vi "_Update A Key Value.vi"(4 "error in (no error)":errorcluster, 5 "Value":string="test Key", 6 "Key":string="Key", 7 "node in":refnum<k20>) -> (0 "error out":errorcluster, 3 "node out":refnum<k20>)   [LabVIEW 2012]
uses:
  <vilib>/xml/Close Reference(Node).vi
  <vilib>/xml/NI_XML.lvlib
  <resource>/objmgr/DOMUserDefRef.rc
panel:
  # "<NameEntry>\n    <Key>old Key</Key>\n    <Name>name value</Name>\n </NameEntry>"
  # "<NameEntry>\n    <Key>test Key</Key>\n    <Name>name value</Name>\n </NameEntry>"
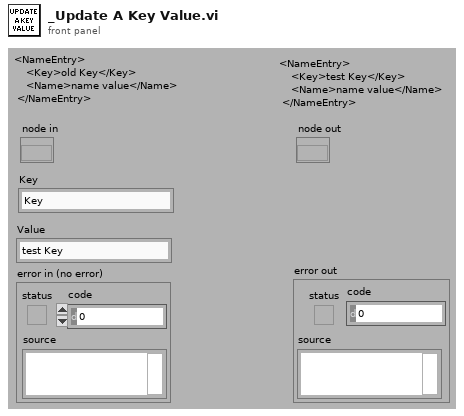
[diagram p1: front panel]
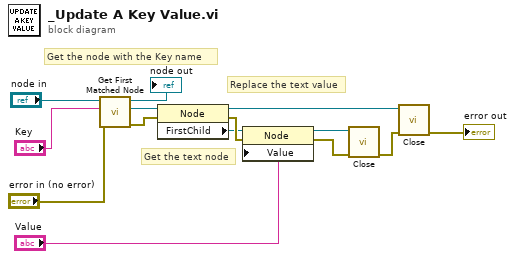
[diagram p0: block diagram]
diagram:
  # "Replace the text value"
  # "Get the text node"
  # "Get the node with the Key name"
  n1 = call <vilib>:"Get First Matched Node.vi"("error in (no error)"="error in (no error)", "XPath expression"="Key", "node in"="node in") -> ("error out"=w8:errorcluster, "node result"=w9:refnum<k20>, "node out"=→"node out":refnum<k20>)  [unwired: 6 in]
  n2 = property class="Node"(reference=w9, error in=w8) -> (reference out=w5:refnum<k20>, error out=w10:errorcluster, "FirstChild"=w7:refnum<k20>)
  n3 = property class="Node"(reference=w7, error in=w10, "Value"="Value") -> (reference out=w2:refnum<k20>, error out=w1:errorcluster)
  n4 = call-poly <vilib>:"Close.vi"("error in (no error)"=w1, "node"=w2) -> ("error out"=w6:errorcluster)  [unwired: 7 in]
  n5 = call-poly <vilib>:"Close.vi"("error in (no error)"=w6, "node"=w5) -> ("error out"=→"error out":errorcluster)  [unwired: 7 in]
